vi "Status - Update cRIO Status.vi"(7 "Skip TimeStamps":bool, 8 "Error In":errorcluster, 9 "[PlantId],[SystemId]":cluster{"[PlantId]":string, "[SystemId]":string}, 11 "cRIO Status":refnum<vi>) -> (0 "Error Out":errorcluster)   [LabVIEW 2013]
uses:
  Controls/DB - [Execute].[ActiveProcess] Enum.ctl
  Controls/DB - CMS Execute Active Process.ctl
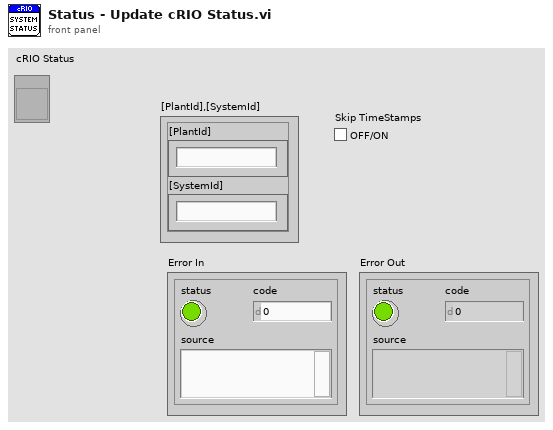
[diagram p1: front panel]
types:
  T1 = typedef "DB - CMS Execute Active Process.ctl" = enum16{"INSERT INTO [Execute].[ActiveProcess]", "UPDATE [Execute].[ActiveProcess]", "SELECT [Execute].[ActiveProcess]", "UPDATE FILESTREAM", "SELECT FILESTREAM", "Check [IsActive]"}
  T2 = typedef "DB - [Execute].[ActiveProcess] Enum.ctl" = enum16{"[IsActive]", "[TransactionNo]", "[TransactionRunNo]", "[SequenceStatus]", "[StartRecordTime]", "[EndRecordTime]", "[StartHoldTime]", "[EndHoldTime]", "[Message1]", "[Message2]", "[HoldTimeRemaining]", "[HoldTimePercentage]", "[HoldProgressColor]", "[OrderNumbers]", "[CurrentTemp]", "[UnitOfTemperature]", "[IsAppClientLive]", "[RawDataFile]", "[RecordedMinutes]", "[FurnaceControlStatus]", "[FurnaceControlColor]", "[ControllerStatus]", "[ControllerColor]", "[IsControllerOnline]", "[ProcessColor]", "[OverallColor]", "[LastUpdatedOn]", "[LastUpdatedCmsTime]", "[Inactive]"}
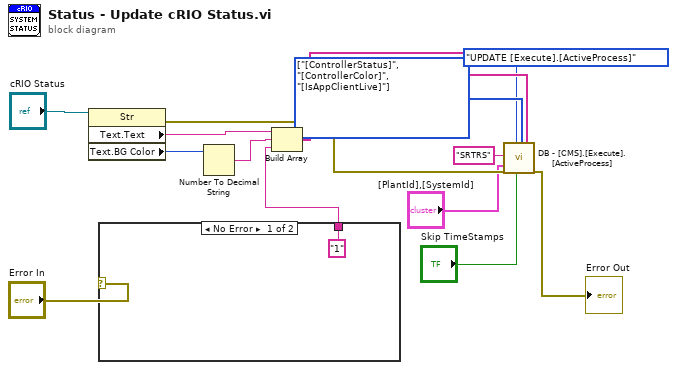
[diagram p0: block diagram]
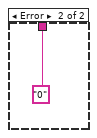
[diagram p2: hidden frame]
diagram:
  w13 = T2[] [enum."[ControllerStatus]", enum."[ControllerColor]", enum."[IsAppClientLive]"] items=["[IsActive]", "[TransactionNo]", "[TransactionRunNo]", "[SequenceStatus]", "[StartRecordTime]", "[EndRecordTime]", "[StartHoldTime]", "[EndHoldTime]", "[Message1]", "[Message2]", "[HoldTimeRemaining]", "[HoldTimePercentage]", "[HoldProgressColor]", "[OrderNumbers]", "[CurrentTemp]", "[UnitOfTemperature]", "[IsAppClientLive]", "[RawDataFile]", "[RecordedMinutes]", "[FurnaceControlStatus]", "[FurnaceControlColor]", "[ControllerStatus]", "[ControllerColor]", "[IsControllerOnline]", "[ProcessColor]", "[OverallColor]", "[LastUpdatedOn]", "[LastUpdatedCmsTime]", "[Inactive]"] ("[Execute].[ActiveProcess]\n2014-10-14 14:58")
  n1 = property class="Str"(reference="cRIO Status") -> (error out=w4:errorcluster, "Text.Text"=w12:string, "Text.BG Color"=w11:u32)  [unwired: 1 in, 1 out]
  n2 = case shown="No Error" "Error In" {
    tunnel: ["1" "0"] -> w8
    frame No Error {
    }
    frame Error {
    }
  }
  n3 = Number To Decimal String(number=w11) -> (decimal integer string=w10:string)  [unwired: 1 in]
  n4 = Build Array(w12, w10, w8) -> (w7:string[])
  n5 = call "DB - [CMS].[Execute].[ActiveProcess].vi"("Application"="SRTRS", "[PlantId],[SystemId]"="[PlantId],[SystemId]", "error in (no error)"=w4, "DB - CMS Execute ActiveProcess"=DB_-_CMS_Execute_Active_Process."UPDATE [Execute].[ActiveProcess]", "Skip TimeStamps"="Skip TimeStamps", "[Execute].[ActiveProcess]\n2014-10-14 14:58"=w13, "<Data>"=w7) -> ("SUMMARY"=→"Error Out":errorcluster)  [unwired: 9 in, 3 out]
